vi "LVCAM Write LVCAM.vi"(10 "LVCAM":refnum<class "LVCAM.lvclass">, 11 "Process in":refnum<class "Process.lvclass">) -> (3 "Process out":refnum<class "Process.lvclass">)   [LabVIEW 2021, in "Process.lvlib" / "Process.lvclass"]
uses:
  Process.lvclass
  LVCAM/LVCAM/LVCAM/LVCAM.lvclass
  Process.lvclass/Process.ctl
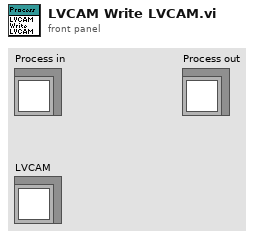
[diagram p1: front panel]
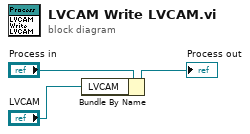
[diagram p0: block diagram]
diagram:
  n1 = Bundle By Name(cluster="Process in", "LVCAM"="LVCAM") -> (→"Process out":refnum<class "Process.lvclass">)
